vi "Read Source path.vi"(9 "Force abs path? (T)":bool=TRUE, 11 "ProjectItem in":refnum<class "ProjectItem.lvclass">) -> (2 "Source path":path, 3 "ProjectItem out":refnum<class "ProjectItem.lvclass">)   [LabVIEW 2019, in "SolutionBuilder.lvlib" / "ProjectItem.lvclass"]
uses:
  ProjectItem.lvclass
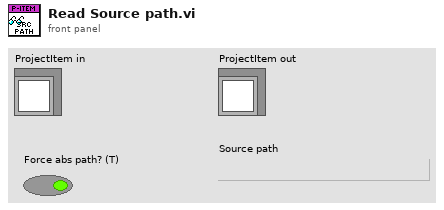
[diagram p1: front panel]
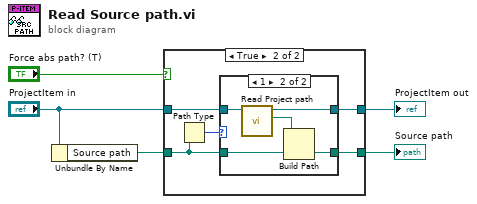
[diagram p0: block diagram]
diagram:
  n1 = Unbundle By Name("ProjectItem in") -> ("Source path"=w2:path)
  n2 = case shown="True" "Force abs path? (T)" {
    tunnel: "ProjectItem in" -> [w7 w12]
    tunnel: [w7 w11] -> w4
    tunnel: w2 -> [w6 w8]
    tunnel: [w6 w9] -> w1
    frame False {
    }
    frame True {
      n3 = Path Type(1:w8) -> (0:w10:i16)
      n4 = case shown="1" w10 {
        tunnel: w12 -> [w14 w19]
        tunnel: [w14 w18] -> w11
        tunnel: [w13 w15] -> w9
        tunnel: w8 -> [w13 w16]
        frame Default {
        }
        frame 1 {
          n5 = call-dynamic "Read Project path.vi"("ProjectItem in"=w19) -> ("Project path"=w17:path, "ProjectItem out"=w18:refnum<class "ProjectItem.lvclass">)  [unwired: 9 in]
          n6 = Build Path(base path=w17, name or relative path=w16) -> (appended path=w15:path)
        }
      }
    }
  }
  "ProjectItem out" <- w4
  "Source path" <- w1
